vi "Configure All Modes.vi"(8 "error in (no error)":errorcluster, 11 "FPGA Interface":refnum<class "FPGA Interface.lvclass">) -> (0 "error out":errorcluster, 3 "1553 Component":refnum<class "1553 Component.lvclass">)   [LabVIEW 2016, in "BCI-1553 RealTime API Examples.lvlib"]
uses:
  BCI-1553 RealTime API Examples.lvlib
  <vilib>/Bloomy/BCI-1553 Driver/RealTime/Dependencies/FPGA Interface/FPGA Interface.lvclass
  <vilib>/Bloomy/BCI-1553 Driver/RealTime/1553 Component/1553 Component.lvclass
  <vilib>/Bloomy/BCI-1553 Driver/RealTime/Bus Controller/Bus Controller.lvclass
  C:/Program Files (x86)/National Instruments/LabVIEW 2016/vi.lib/Bloomy/BCI-1553 Driver/RealTime/1553 SubComponent/1553 SubComponent.lvclass
  <vilib>/Bloomy/BCI-1553 Driver/RealTime/Remote Terminal/Remote Terminal.lvclass
  <vilib>/Bloomy/BCI-1553 Driver/RealTime/Bus Monitor/Bus Monitor.lvclass
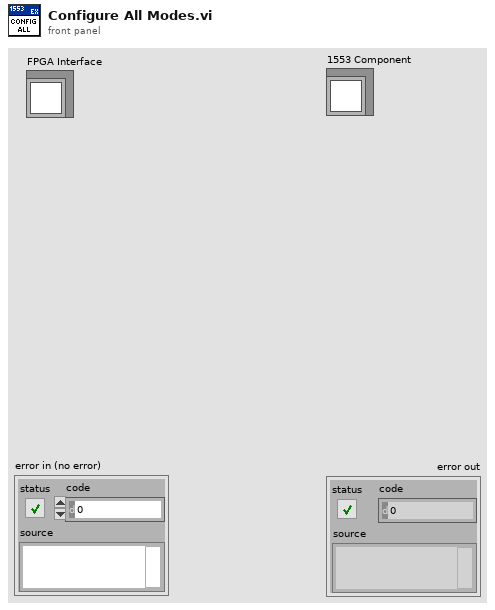
[diagram p1: front panel]
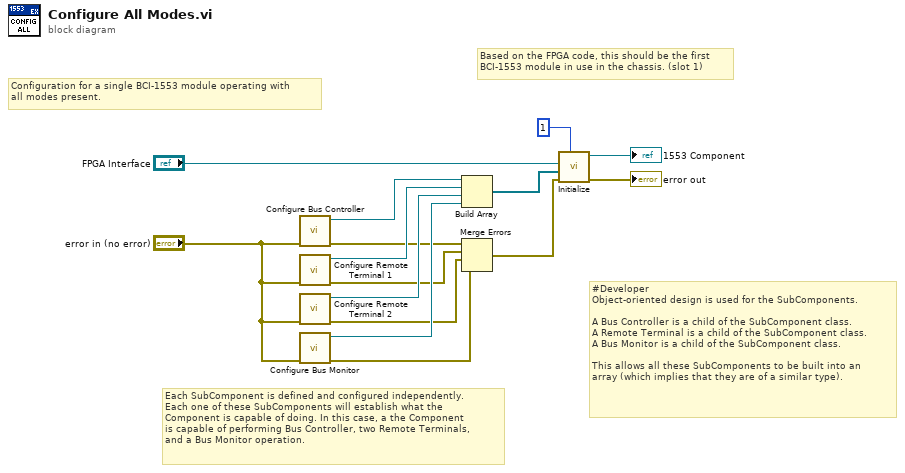
[diagram p0: block diagram]
diagram:
  # "#Developer\nObject-oriented design is used for the SubComponents.\n\nA Bus Controller is a child of the SubComponent class.\nA Remote Terminal is a child of the SubComponent class.\nA Bus Monitor is a child of the SubComponent class.\n\nThis allows all these SubComponents to be built into an\narray (which implies that they are of a similar type)."
  # "Each SubComponent is defined and configured independently.\nEach one of these SubComponents will establish what the\nComponent is capable of doing. In this case, a the Component \nis capable of performing Bus Controller, two Remote Terminals, \nand a Bus Monitor operation."
  # "Configuration for a single BCI-1553 module operating with\nall modes present."
  # "Based on the FPGA code, this should be the first\nBCI-1553 module in use in the chassis. (slot 1)"
  n1 = call "Configure Bus Controller.vi"("error in (no error)"="error in (no error)") -> ("error out"=w5:errorcluster, "Bus Controller"=w11:refnum<class "Bus Controller.lvclass">)  [unwired: 9 in]
  n2 = call "Configure Remote Terminal 1.vi"("error in (no error)"="error in (no error)") -> ("error out"=w4:errorcluster, "Remote Terminal"=w10:refnum<class "Remote Terminal.lvclass">)  [unwired: 9 in]
  n3 = call "Configure Remote Terminal 2.vi"("error in (no error)"="error in (no error)") -> ("error out"=w3:errorcluster, "Remote Terminal"=w9:refnum<class "Remote Terminal.lvclass">)  [unwired: 9 in]
  n4 = call "Configure Bus Monitor.vi"("error in (no error)"="error in (no error)") -> ("error out"=w2:errorcluster, "Bus Monitor"=w8:refnum<class "Bus Monitor.lvclass">)  [unwired: 9 in]
  n5 = Build Array(w11, w10, w9, w8) -> (w7:refnum<class "1553 SubComponent.lvclass">[])
  n6 = Merge Errors(w5, w4, w3, w2) -> (w1:errorcluster)
  n7 = call <vilib>:"Initialize.vi"("Component ID (1-8)"=u8 1, "error in (no error)"=w1, "SubComponents"=w7, "FPGA Interface"="FPGA Interface") -> ("error out"=→"error out":errorcluster, "1553 Component out"=→"1553 Component":refnum<class "1553 Component.lvclass">)  [unwired: 6 in]
